vi "Diagnostics.Protocol.Initialize.vi"(8 "error in (no error)":errorcluster, 11 "Parameters":T6={"Name"="", "CAN"={"Interface"="", "Baud Rate"=0, "Diagnostic Protocol"=enum."GMLAN", "Transport Protocol"=enum."ISO TP - Normal Mode", "Transmit ID"=0, "Receive ID"=0, "Transmit Extension"=0, "Receive Extension"=0, "Receive UUDT ID"=0, "Enable Stream"=FALSE, "VW TP Channel ID"=1, "Fill Frame"=FALSE, "Fill Byte"=0, "Termination"=FALSE, "LIN Cluster"="", "NAD"=8, "IO Mode"=0, "Max DLC"=0, "FD Baud Rate"=0, "Timeout"=0, "FD ISO Mode"=0, "DoIP Address"="", "DoIP Source Address"=3584, "DoIP Dynamic Port"=TRUE, "DoIP Version"=2}, "986x"={"Enable"=FALSE, "RIO Device"="", "Bitfile"=path ""}, "Reads"=[], "Frames Lookup"=variant, "Writes"=[], "DPIDs"=[], "DPID Lookup"=variant, "DTC"={"Descriptor"={"DTC Byte Length"=0, "Status Byte Length"=1, "Add Data Byte Length"=1, "Byte Order"=enum."Motorola"}, "Value.Code"=[], "Value.String"=[], "Value.J2012String"=[], "Status.Code"=[], "Status.String"=[]}, "Created DTCs"=0, "Polls"=[], "Service Channels Status Lookup"=variant, "Trigger Lookup"=variant, "Security"={"Type"=enum."None", "Source DLL Path"=path "", "Target DLL Path"=path "", "Security Level"=0, "Static Master Key"="", "Max Key Length"=1, "Host IP Address"="", "ECU  Variant"=0, "Optional Parameter"=0}, "Initial Comm State"=FALSE} {"Writes"."Signals"."Byte Order" items=["Little Endian", "Big Endian"]; "Writes"."Signals"."Data Type" items=["Signed", "Unsigned", "IEEE Float"]; "CAN"."DoIP Version" items=["2010"=1, "2012"=2]; "CAN"."DoIP Source Address" format="%.0x"; "CAN"."FD ISO Mode" items=["ISO", "Non ISO", "ISO Legacy"]; "CAN"."IO Mode" items=["CAN 2.0", "CAN FD", "CAN FD+BRS"]; "CAN"."Fill Byte" format="%.0x"; "CAN"."VW TP Channel ID" format="%.0x"; "CAN"."Receive UUDT ID" format="%.0x"; "CAN"."Receive Extension" format="%.0x"; "CAN"."Transmit Extension" format="%.0x"; "CAN"."Receive ID" format="%.0x"; "CAN"."Transmit ID" format="%.0x"; "Reads"."Signals"."Byte Order" items=["Little Endian", "Big Endian"]; "Reads"."Signals"."Data Type" items=["Signed", "Unsigned", "IEEE Float"]}) -> (0 "error out":errorcluster, 3 "diag ref out":T1={"Diag CAN Handle"=0, "Transport Protocol"=enum."ISO TP - Normal Mode", "Receive Address Extension"=0, "Transmit Address Extension"=0, "Receive CAN Id"=0, "Transmit CAN Id"=0, "Log Frames ?"=FALSE, "My TP Address"=0, "Other TP Address"=0, "T1"=0, "T2"=0, "T3"=0, "T4"=0, "Tx SN"=0, "Block Size"=0, "Rx SN"=0, "VW TP Initialized?"=FALSE, "Tx block no"=0, "baud rate"=0, "Interface"="", "Channel Diag CAN Handle"=0, "UDP Connection ID"=refnum, "TCP Connection ID"=refnum, "Target IP Addr"=0, "Source Address"=0, "Target Address"=0, "Send Header NACK?"=FALSE, "DLL Handle"=0, "NAD"=0, "Time Stamp read first"=0.0, "Time Stamp read last"=0.0, "Time Stamp write first"=0.0, "Time Stamp write last"=0.0, "Time Stamp write"=0.0, "Time Stamp read"=0.0, " I/O Mode"=0, "FD Baudrate"=0, "TX_DL"=8, "RX_DL"=8, "DoIP Protocol Version"=1, " Selected I/O Mode"=0, "TesterPresent Counter"=0, "TesterPresent Limit"=0, "TesterPresent Tick[ms]"=10, "TesterPresent RequireResponse?"=FALSE, "TesterPresent Stored Ref?"=FALSE, "TesterPresent Message"=[], "TesterPresent Task Handle"=0, "TesterPresent Semaphore"=refnum, "Response Plausibility Check"=1, "Default Version?"=TRUE, "Diagostic Globals"={"Timeout FC (Bs)"=250, "Timeout CF (Cr)"=250, "Timeout Diag Command"=1000, "Receive Block Size (BS)"=0, "Wait Time CF (STmin)"=5, "Max Waits (N_WFTmax)"=10, "Waits to Send (N_WAIT)"=0, "Time between Waits (TW)"=25, "Fill CAN Frames?"=TRUE, "Fill Byte"=255, "Invalid Response as Error?"=FALSE, "Max RspPending Count"=5, "VWTP Command Timeout"=50, "Transport Protocol"=enum."Diagnostics on IP", "Diag CAN Handle"=0, "DLL Handle"=0, "Timeout RspPending"=1000}, "Session-based Properties?"=FALSE, "NI-XNET IP Stack Reference"=0, "NI-XNET IP Stack TCP Reference"=-1, "NI-XNET IP Stack UDP Reference"=-1, "NI-XNET IP Stack Local Interface"="", "Functional CAN Id"=0, "Diag CAN Queue"=refnum, "Frame Fillling Mode"=0, "DoIP Acknowledge Mode"=0, "Message Buffer"=[]} {"Diagostic Globals"."Fill Byte" format="%x"; "TesterPresent Message" format="%.0x"; "Selected I/O Mode" items=["CAN", "CAN FD", "CAN FD+BRS", "ECU Determined"]; "DoIP Protocol Version" items=["2010"=1, "2012"=2]; "RX_DL" items=["8"=8, "12"=12, "16"=16, "20"=20, "24"=24, "32"=32, "48"=48, "64"=64]; "TX_DL" items=["8"=8, "12"=12, "16"=16, "20"=20, "24"=24, "32"=32, "48"=48, "64"=64]; "I/O Mode" items=["CAN", "CAN FD", "CAN FD+BRS", "Not yet determined"]})   [LabVIEW 2024, in "Diagnostics Addon Engine.lvlib"]
uses:
  Diagnostics Addon Engine.lvlib
  Addon Shared/Types/SysDef.Compile.ctl
  Addon Shared/Types/CAN.ctl
  Addon Shared/Types/CAN.Interface.ctl
  Addon Shared/Types/Protocol.ctl
  Addon Shared/Types/Transport.ctl
  Addon Shared/Types/986x.ctl
  Addon Shared/Types/Frame.Compile.ctl
  Addon Shared/Types/Type.ctl
  Addon Shared/Types/Signal.ctl
  Addon Shared/Types/DPID.ctl
  Addon Shared/Types/DPID.Rate.ctl
  Addon Shared/Types/DTC.Settings.ctl
  Addon Shared/Types/DTC.Descriptor.ctl
  Addon Shared/Types/Poll.Compiled.ctl
  Addon Shared/Types/Security.ctl
  Addon Shared/Types/Security.Type.ctl
  <vilib>/Automotive Diagnostic Command Set/Diagnostic Transport.llb/Diag Reference.ctl
  <vilib>/Automotive Diagnostic Command Set/Diagnostic Transport.llb/Transport Protocol Selector.ctl
  <vilib>/Automotive Diagnostic Command Set/Diagnostic Transport.llb/DoIP Protocol Version.ctl
  <vilib>/Automotive Diagnostic Command Set/Diagnostic Transport.llb/Diag Globals.ctl
  <vilib>/Automotive Diagnostic Command Set/Diagnostic Transport.llb/Property ID.ctl
  <vilib>/Automotive Diagnostic Command Set/Diagnostic Transport.llb/VWTP Application Type.ctl
  <vilib>/addons/Automotive Diagnostic Command Set/NI_Automotive Diagnostic Command Set.lvlib
  Addon Shared/Diagnostics Addon Shared.lvlib
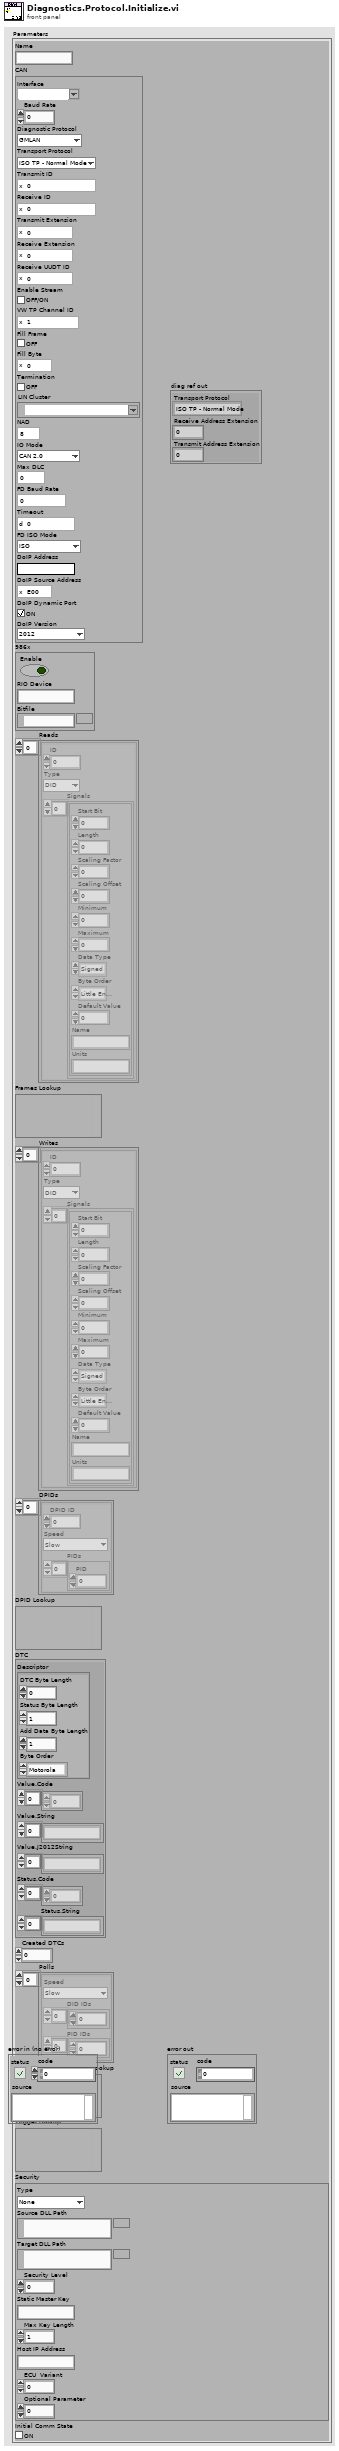
[diagram p1: front panel]
types:
  T1 = typedef "NI_Automotive Diagnostic Command Set.lvlib/Diag Reference.ctl" = cluster{"Diag CAN Handle":u32, "Transport Protocol":T2, "Receive Address Extension":u8, "Transmit Address Extension":u8, "Receive CAN Id":u32, "Transmit CAN Id":u32, "Log Frames ?":bool, "My TP Address":u8, "Other TP Address":u8, "T1":u16, "T2":u16, "T3":u16, "T4":u16, "Tx SN":u8, "Block Size":u8, "Rx SN":u8, "VW TP Initialized?":bool, "Tx block no":u8, "baud rate":u64, "Interface":string, "Channel Diag CAN Handle":u32, "UDP Connection ID":refnum<k16>, "TCP Connection ID":refnum<k5>, "Target IP Addr":u32, "Source Address":u16, "Target Address":u16, "Send Header NACK?":bool, "DLL Handle":u32, "NAD":u8, "Time Stamp read first":dbl, "Time Stamp read last":dbl, "Time Stamp write first":dbl, "Time Stamp write last":dbl, "Time Stamp write":dbl, "Time Stamp read":dbl, " I/O Mode":u32, "FD Baudrate":u64, "TX_DL":u16, "RX_DL":u16, "DoIP Protocol Version":T3, " Selected I/O Mode":u32, "TesterPresent Counter":u32, "TesterPresent Limit":u32, "TesterPresent Tick[ms]":i32, "TesterPresent RequireResponse?":bool, "TesterPresent Stored Ref?":bool, "TesterPresent Message":u8[], "TesterPresent Task Handle":i32, "TesterPresent Semaphore":T4, "Response Plausibility Check":u32, "Default Version?":bool, "Diagostic Globals":T5, "Session-based Properties?":bool, "NI-XNET IP Stack Reference":i64, "NI-XNET IP Stack TCP Reference":i64, "NI-XNET IP Stack UDP Reference":i64, "NI-XNET IP Stack Local Interface":string, "Functional CAN Id":u32, "Diag CAN Queue":refnum<queue>, "Frame Fillling Mode":u32, "DoIP Acknowledge Mode":u32, "Message Buffer":u8[]}
  T2 = typedef "NI_Automotive Diagnostic Command Set.lvlib/Transport Protocol Selector.ctl" = enum16{"ISO TP - Normal Mode", "ISO TP - Mixed Mode", "VW TP 2.0", "Diagnostics on IP", "ISO TP LIN"}
  T3 = typedef "NI_Automotive Diagnostic Command Set.lvlib/DoIP Protocol Version.ctl" = u8
  T4 = typedef "Semaphore RefNum" = refnum<k1>
  T5 = typedef "NI_Automotive Diagnostic Command Set.lvlib/Diag Globals.ctl" = cluster{"Timeout FC (Bs)":u32, "Timeout CF (Cr)":u32, "Timeout Diag Command":u32, "Receive Block Size (BS)":u8, "Wait Time CF (STmin)":u8, "Max Waits (N_WFTmax)":u8, "Waits to Send (N_WAIT)":i32, "Time between Waits (TW)":u32, "Fill CAN Frames?":bool, "Fill Byte":u32, "Invalid Response as Error?":bool, "Max RspPending Count":u32, "VWTP Command Timeout":u32, "Transport Protocol":T2, "Diag CAN Handle":u32, "DLL Handle":u32, "Timeout RspPending":u32}
  T6 = typedef "Diagnostics Addon Shared.lvlib/SysDef.Compile.ctl" = cluster{"Name":string, "CAN":T7, "986x":T11, "Reads":T12[], "Frames Lookup":variant, "Writes":T12[], "DPIDs":T15[], "DPID Lookup":variant, "DTC":T17, "Created DTCs":u32, "Polls":T19[], "Service Channels Status Lookup":variant, "Trigger Lookup":variant, "Security":T20, "Initial Comm State":bool}
  T7 = typedef "Diagnostics Addon Shared.lvlib/CAN.ctl" = cluster{"Interface":T8, "Baud Rate":u64, "Diagnostic Protocol":T9, "Transport Protocol":T10, "Transmit ID":u32, "Receive ID":u32, "Transmit Extension":u8, "Receive Extension":u8, "Receive UUDT ID":u32, "Enable Stream":bool, "VW TP Channel ID":u32, "Fill Frame":bool, "Fill Byte":u8, "Termination":bool, "LIN Cluster":refnum<k21>, "NAD":u8, "IO Mode":u32, "Max DLC":u16, "FD Baud Rate":u64, "Timeout":u32, "FD ISO Mode":u32, "DoIP Address":string, "DoIP Source Address":u16, "DoIP Dynamic Port":bool, "DoIP Version":u16}
  T8 = typedef "Diagnostics Addon Shared.lvlib/CAN.Interface.ctl" = string
  T9 = typedef "Diagnostics Addon Shared.lvlib/Protocol.ctl" = enum16{"GMLAN", "KWP-2000", "UDS", "User-Defined"}
  T10 = typedef "Diagnostics Addon Shared.lvlib/Transport.ctl" = enum16{"ISO TP - Normal Mode", "ISO TP - Mixed Mode", "VW TP 2.0", "Diagnostics on IP", "ISO TP LIN"}
  T11 = typedef "Diagnostics Addon Shared.lvlib/986x.ctl" = cluster{"Enable":bool, "RIO Device":string, "Bitfile":path}
  T12 = typedef "Diagnostics Addon Shared.lvlib/Frame.Compile.ctl" = cluster{"ID":u32, "Type":T13, "Signals":T14[]}
  T13 = typedef "Diagnostics Addon Shared.lvlib/Type.ctl" = enum16{"DID", "CDID", "PID", "CPID", "Read Memory", "Write Memory", "IO Control", "Routine Start", "Routine Request", "Routine Stop", "User Defined", "DTC Control", "Clear DTCs", "Read DTCs", "Start DTCs", "DTC Change Count", "Tester Present", "Unlock ECU", "Reset ECU", "Diag Session Control", "Communication Control", "DPID Control", "Poll Control", "Diag Comm Port Control"}
  T14 = typedef "Diagnostics Addon Shared.lvlib/Signal.ctl" = cluster{"Start Bit":u32, "Length":u32, "Scaling Factor":dbl, "Scaling Offset":dbl, "Minimum":dbl, "Maximum":dbl, "Data Type":u32, "Byte Order":u32, "Default Value":dbl, "Name":string, "Units":string}
  T15 = typedef "Diagnostics Addon Shared.lvlib/DPID.ctl" = cluster{"DPID ID":u8, "Speed":T16, "PIDs":u16[]}
  T16 = typedef "Diagnostics Addon Shared.lvlib/DPID.Rate.ctl" = enum16{"Slow", "Medium", "Fast"}
  T17 = typedef "Diagnostics Addon Shared.lvlib/DTC.Settings.ctl" = cluster{"Descriptor":T18, "Value.Code":dbl[], "Value.String":string[], "Value.J2012String":string[], "Status.Code":dbl[], "Status.String":string[]}
  T18 = typedef "Diagnostics Addon Shared.lvlib/DTC.Descriptor.ctl" = cluster{"DTC Byte Length":i32, "Status Byte Length":i32, "Add Data Byte Length":i32, "Byte Order":enum16{"Motorola", "Intel"}}
  T19 = typedef "Diagnostics Addon Shared.lvlib/Poll.Compiled.ctl" = cluster{"Speed":T16, "DID IDs":u32[], "PID IDs":u32[]}
  T20 = typedef "Diagnostics Addon Shared.lvlib/Security.ctl" = cluster{"Type":T21, "Source DLL Path":path, "Target DLL Path":path, "Security Level":u32, "Static Master Key":string, "Max Key Length":u32, "Host IP Address":string, "ECU  Variant":i8, "Optional Parameter":i8}
  T21 = typedef "Diagnostics Addon Shared.lvlib/Security.Type.ctl" = enum16{"None", "SeedKey DLL", "MasterKey (Channel)", "MasterKey (Static)", "SeedKey DLL (Windows)"}
  T22 = typedef "NI_Automotive Diagnostic Command Set.lvlib/Property ID.ctl" = enum16{"Timeout Diag Command", "Timeout FC (Bs)", "Timeout CF (Cr)", "Receive Block Size (BS)", "Wait Time CF (STmin)", "Max Wait Frames (N_WFTmax)", "Wait Frames to Send (N_WAIT)", "Time between Waits (T_W)", "Fill CAN Frames", "Fill Byte", "Invalid Response as Error", "Max RspPending Count", "VWTP Command Timeout", "STmin", "P2min", "Termination", "Timeout RspPending", "LIN Sleep", "Actual CAN IO Mode", "Response Plausibility Check", "Session-based Properties", "DoIP Acknowledge Mode"}
  T23 = typedef "NI_Automotive Diagnostic Command Set.lvlib/VWTP Application Type.ctl" = u8
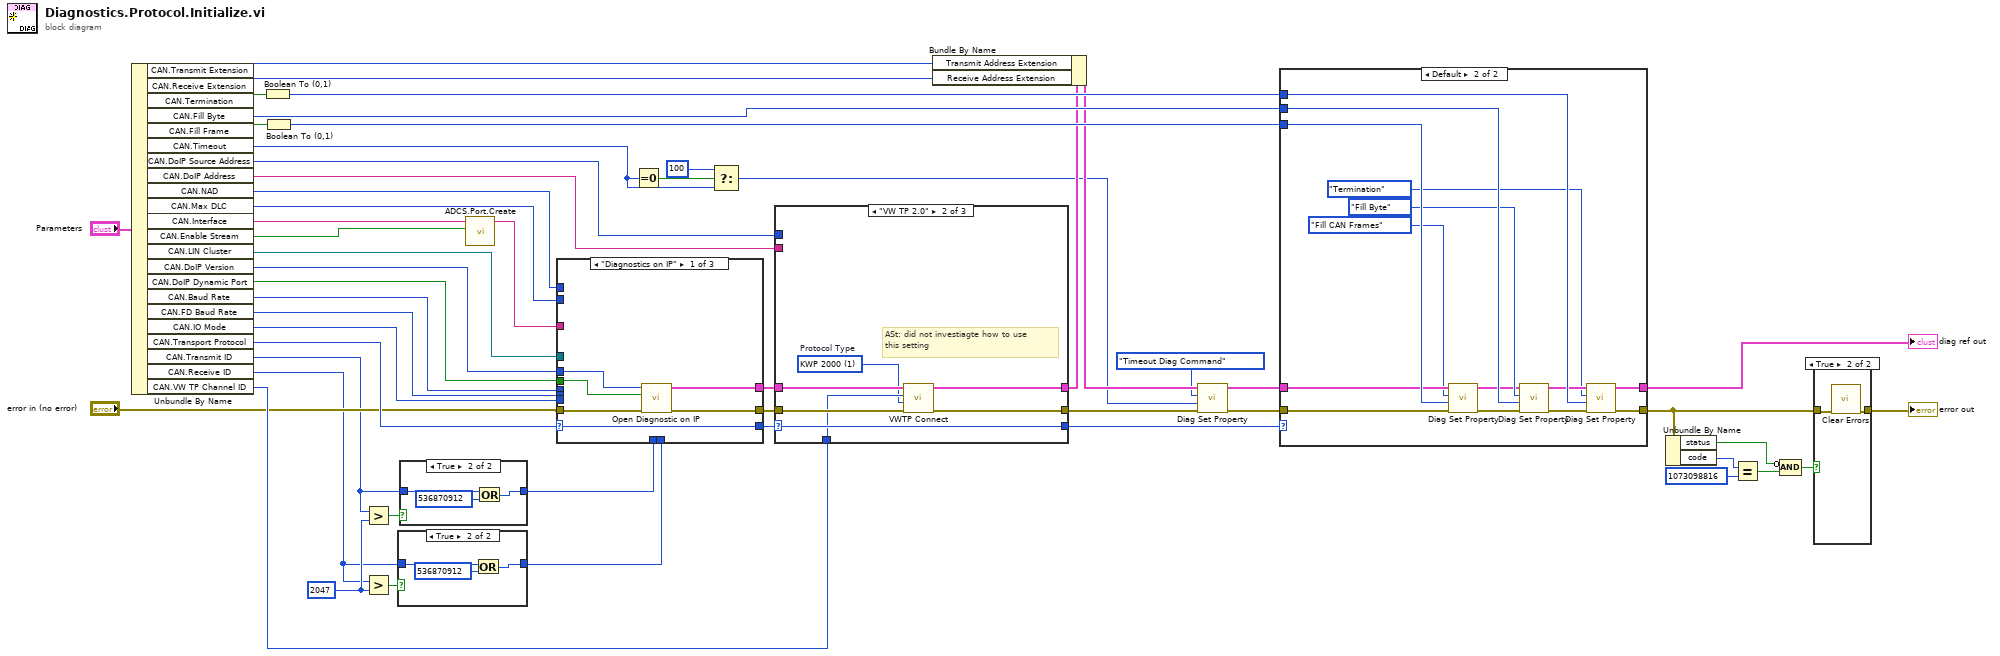
[diagram p0: block diagram]
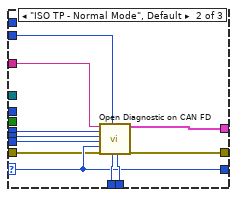
[diagram p5: hidden frame]
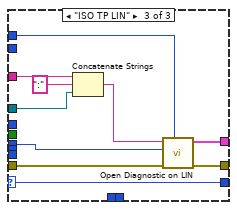
[diagram p6: hidden frame]
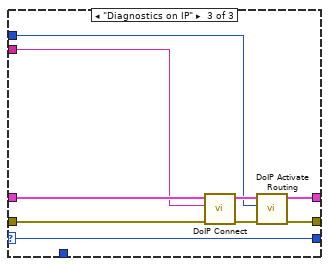
[diagram p9: hidden frame]
diagram:
  w29 = u32 2047 ("y")
  n1 = Unbundle By Name("Parameters") -> ("CAN.Transmit Extension"=w31:u8, "CAN.Receive Extension"=w32:u8, "CAN.Termination"=w49:bool, "CAN.Fill Byte"=w47:u8, "CAN.Fill Frame"=w48:bool, "CAN.Timeout"=w15:u32, "CAN.DoIP Source Address"=w1:u16, "CAN.DoIP Address"=w5:string, "CAN.NAD"=w22:u8, "CAN.Max DLC"=w21:u16, "CAN.Interface"=w30:T8, "CAN.Enable Stream"=w18:bool, "CAN.LIN Cluster"=w17:refnum<k21>, "CAN.DoIP Version"=w3:u16, "CAN.DoIP Dynamic Port"=w2:bool, "CAN.Baud Rate"=w53:u64, "CAN.FD Baud Rate"=w20:u64, "CAN.IO Mode"=w19:u32, "CAN.Transport Protocol"=w35:T10, "CAN.Transmit ID"=w26:u32, "CAN.Receive ID"=w24:u32, "CAN.VW TP Channel ID"=w42:u32)
  n2 = Boolean To (0,1)(Boolean=w49) -> (0, 1=w50:i16)
  n3 = Boolean To (0,1)(Boolean=w48) -> (0, 1=w51:i16)
  n4 = Greater?(x=w26, y=w29) -> (0:w28:bool)
  n5 = Greater?(x=w24, y=w29) -> (0:w27:bool)
  n6 = case shown="True" w27 {
    tunnel: w24 -> [w54 w56]
    tunnel: [w54 w55] -> w23
    frame False {
    }
    frame True {
      n7 = Or(x=w56, y=u32 536870912) -> (x .or. y?=w55:u32)
    }
  }
  n8 = case shown="True" w28 {
    tunnel: w26 -> [w58 w61]
    tunnel: [w58 w60] -> w25
    frame False {
    }
    frame True {
      n9 = Or(x=w61, y=u32 536870912) -> (x .or. y?=w60:u32)
    }
  }
  n10 = call "ADCS.Port.Create.vi"("Enable Stream"=w18, "CAN port"=w30) -> ("CAN port out"=w37:string)  [unwired: 9 in]
  n11 = case shown="\"Diagnostics on IP\"" w35 {
    selector: w35 -> [w67 w73 w88]
    tunnel: w25 -> [_ w78 _]
    tunnel: w53 -> [_ w77 w86]
    tunnel: w23 -> [_ w76 _]
    tunnel: [w65 w75 w85] -> w38
    tunnel: [w66 w68 w84] -> w40
    tunnel: w37 -> [_ w74 w80]
    tunnel: [w67 w73 w88] -> w36
    tunnel: "error in (no error)" -> [w64 w72 w87]
    tunnel: w22 -> [_ _ w83]
    tunnel: w21 -> [_ w71 _]
    tunnel: w20 -> [_ w70 _]
    tunnel: w19 -> [_ w69 _]
    tunnel: w17 -> [_ _ w81]
    tunnel: w3 -> [w63 _ _]
    tunnel: w2 -> [w62 _ _]
    frame "Diagnostics on IP" {
      n12 = call <vilib>:"Open Diagnostic on IP.vi"("error in (no error)"=w64, "dynamic port?"=w62, "protocol version"=w63) -> ("error out"=w66:errorcluster, "Diag reference out"=w65:T1)  [unwired: 3 in, 4 out]
    }
    frame "ISO TP - Normal Mode", Default {
      n13 = call <vilib>:"Open Diagnostic on CAN FD.vi"("CAN Interface"=w74, "Baud Rate"=w77, "FD Baud Rate"=w70, "IO Mode"=w69, "Transport Protocol"=w73, "error in (no error)"=w72, "Max DLC"=w71, "Transmit ID"=w78, "Receive ID"=w76) -> ("diag ref out"=w75:T1, "error out"=w68:errorcluster)  [unwired: 9 in]
    }
    frame "ISO TP LIN" {
      n14 = Concatenate Strings(w80, ":" ("string"), w81) -> (w79:string)
      n15 = call <vilib>:"Open Diagnostic on LIN.vi"("NAD"=w83, "error in (no error)"=w87, "Baud Rate"=w86, "Interface"=w79) -> ("error out"=w84:errorcluster, "Diag Ref Out"=w85:T1)  [unwired: 6 in]
    }
  }
  n16 = Equal To 0?(x=w15) -> (x = 0?=w16:bool)
  n17 = Select(t=u32 100, s=w16, f=w15) -> (s? t:f=w13:u32)
  n18 = case shown="\"VW TP 2.0\"" w36 {
    selector: w36 -> [w91 w96 w103]
    tunnel: [w90 w98 w106] -> w39
    tunnel: [w89 w97 w104] -> w41
    tunnel: [w91 w96 w103] -> w4
    tunnel: w38 -> [w90 w95 w101]
    tunnel: w40 -> [w89 w94 w102]
    tunnel: w42 -> [_ w93 _]
    tunnel: w5 -> [_ _ w100]
    tunnel: w1 -> [_ _ w99]
    frame "ISO TP - Normal Mode", Default {
    }
    frame "VW TP 2.0" {
      w92 = T23 1 items=["KWP 2000"=1, "KS Type 010C"=2, "Infotainment communication"=16, "Application protocol"=32, "WFS/WIV"=33]  # Protocol Type
      # "ASt: did not investiagte how to use\nthis setting"
      n19 = call <vilib>:"VWTP Connect.vi"("error in"=w94, "application type"=w92, "channel ID"=w93, "diag ref in"=w95) -> ("error out"=w97:errorcluster, "diag ref out"=w98:T1)  [unwired: 6 out]
    }
    frame "Diagnostics on IP" {
      n20 = call <vilib>:"DoIP Connect.vi"("error in (no error)"=w102, "address"=w100, "Diag Reference in"=w101) -> ("error out"=w105:errorcluster, "Diag reference out"=w107:T1)  [unwired: 5 in, 2 out]
      n21 = call <vilib>:"DoIP Activate Routing.vi"("error in (no error)"=w105, "Source Address"=w99, "Diag reference in"=w107) -> ("error out"=w104:errorcluster, "Diag reference out"=w106:T1)  [unwired: 1 in, 6 out]
    }
  }
  n22 = Bundle By Name(cluster=w39, "Transmit Address Extension"=w31, "Receive Address Extension"=w32) -> (w43:T1)
  n23 = call <vilib>:"Diag Set Property.vi"("error in (no error)"=w41, "property value"=w13, "property ID"=Property_ID."Timeout Diag Command", "diag ref in"=w43) -> ("error out"=w44:errorcluster, "diag ref out"=w45:T1)  [unwired: 6 in]
  n24 = case shown="Default" w4 {
    tunnel: w51 -> [_ w123]
    tunnel: w50 -> [_ w122]
    tunnel: w47 -> [_ w121]
    tunnel: [w108 w120] -> w46
    tunnel: w45 -> [w108 w118]
    tunnel: w44 -> [w109 w114]
    tunnel: [w109 w110] -> w7
    frame "Diagnostics on IP" {
    }
    frame Default {
      n25 = call <vilib>:"Diag Set Property.vi"("error in (no error)"=w114, "property value"=w123, "property ID"=Property_ID."Fill CAN Frames", "diag ref in"=w118) -> ("error out"=w112:errorcluster, "diag ref out"=w111:T1)  [unwired: 6 in]
      n26 = call <vilib>:"Diag Set Property.vi"("error in (no error)"=w112, "property value"=w121, "property ID"=Property_ID."Fill Byte", "diag ref in"=w111) -> ("error out"=w113:errorcluster, "diag ref out"=w119:T1)  [unwired: 6 in]
      n27 = call <vilib>:"Diag Set Property.vi"("error in (no error)"=w113, "property value"=w122, "property ID"=Property_ID."Termination", "diag ref in"=w119) -> ("error out"=w110:errorcluster, "diag ref out"=w120:T1)  [unwired: 6 in]
    }
  }
  "diag ref out" <- w46
  n28 = Unbundle By Name(w7) -> ("status"=w9:bool, "code"=w12:i32)
  n29 = Equal?(x=w12, y=1073098816) -> (x = y?=w10:bool)
  n30 = Compound Arithmetic op=AND(invert w9, w10) -> (w8:bool)
  n31 = case shown="True" w8 {
    tunnel: w7 -> [w124 w126]
    tunnel: [w124 w125] -> w6
    frame False {
    }
    frame True {
      n32 = call <vilib>:"Clear Errors.vi"("error in (no error)"=w126) -> ("error out"=w125:errorcluster)  [unwired: 5 in, 1 out]
    }
  }
  "error out" <- w6
